vi "AppendWaveformArray.vi"(10 "Array B":waveform(dbl)[](array[waveform]), 11 "Array A":waveform(dbl)[](array[waveform])) -> (3 "Array out":waveform(dbl)[](array[waveform]))   [LabVIEW 2013]
uses:
  <vilib>/Waveform/WDTOps.llb/WDT Append Waveforms DBL.vi
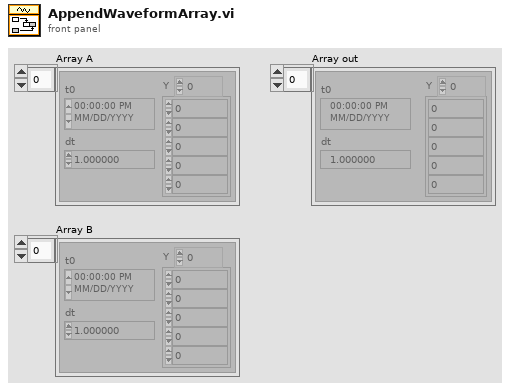
[diagram p1: front panel]
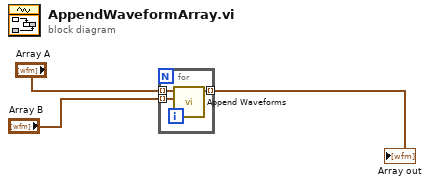
[diagram p0: block diagram]
diagram:
  n1 = for {
    tunnel: "Array B" -> [w6] mode=indexing
    tunnel: "Array A" -> [w5] mode=indexing
    tunnel: [w4] -> w3 mode=indexing
    n2 = call-poly <vilib>:"Append Waveforms.vi"("waveform B"=w6, "waveform A"=w5) -> ("waveform out"=w4:waveform(dbl))  [unwired: 8 in, 1 out]
  }
  "Array out" <- w3
